vi "Write Array of Launch Instrument Addresses.vi"(8 "error in (no error)":errorcluster, 10 "Array of Launch Instrument Addresses":refnum<class "Message Enqueuer.lvclass">[](array[class]), 11 "Instrument Finder in":refnum<class "Instrument Finder.lvclass">) -> (0 "error out":errorcluster, 3 "Instrument Finder out":refnum<class "Instrument Finder.lvclass">)   [LabVIEW 2014, in "SetUp VIs.lvlib" / "Instrument Finder.lvclass"]
uses:
  Instrument Finder.lvclass
  <vilib>/ActorFramework/Message Enqueuer/Message Enqueuer.lvclass
  Instrument Finder.lvclass/Instrument Finder.ctl
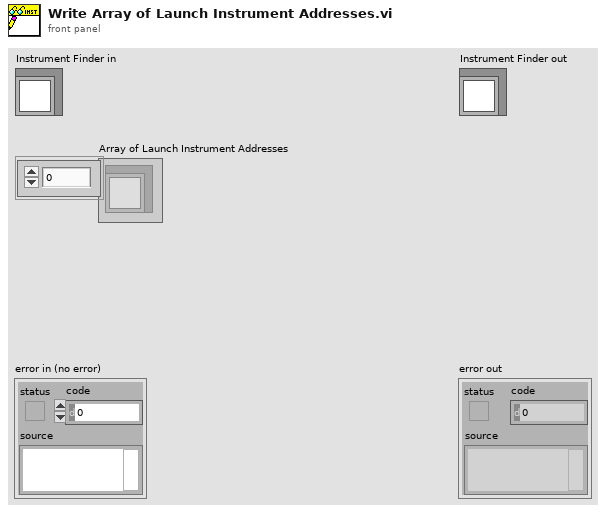
[diagram p1: front panel]
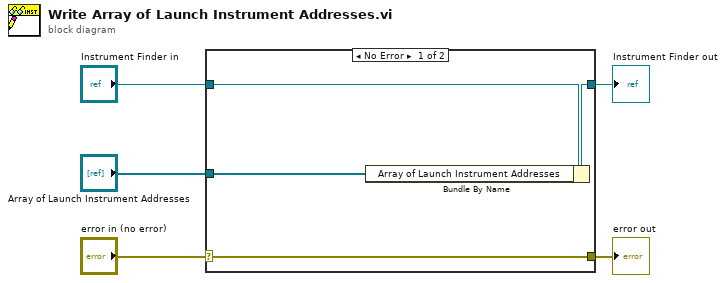
[diagram p0: block diagram]
diagram:
  n1 = case shown="No Error" "error in (no error)" {
    selector: "error in (no error)" -> [w9 w10]
    tunnel: [w9 w10] -> w4
    tunnel: [w7 w11] -> w2
    tunnel: "Instrument Finder in" -> [w8 w11]
    tunnel: "Array of Launch Instrument Addresses" -> [w6 _]
    frame No Error {
      n2 = Bundle By Name(cluster=w8, "Array of Launch Instrument Addresses"=w6) -> (w7:refnum<class "Instrument Finder.lvclass">)
    }
    frame Error {
    }
  }
  "error out" <- w4
  "Instrument Finder out" <- w2
